vi "UDP广播.vi"(4 "接收间隔(5ms)":u32=5, 6 "发送间隔(25ms)":u32=25, 7 "文本控件":refnum<vi>, 8 "错误输入（无错误）":errorcluster, 10 "数据输入":string="www.usr.cn", 11 "端口或服务名称":u16=48899) -> (0 "error out":errorcluster caption="错误输出", 3 "接收":string[](array[string])=["192.168.1.221,D8B04CECA550,USR-C215,2.2.6", "192.168.1.220,ACCF2363AFF8,"])   [LabVIEW 2017]
uses:
  f306e6eb-da80-433f-8739-1ff3909e1865.vi
panel:
  out "发送次数":i32
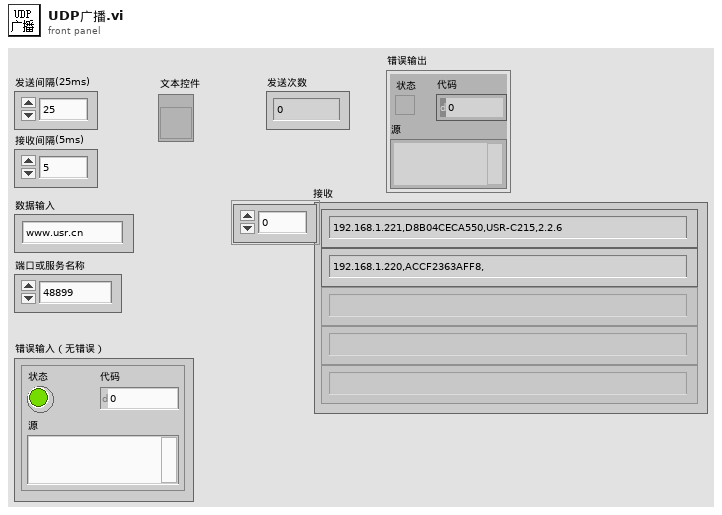
[diagram p1: front panel]
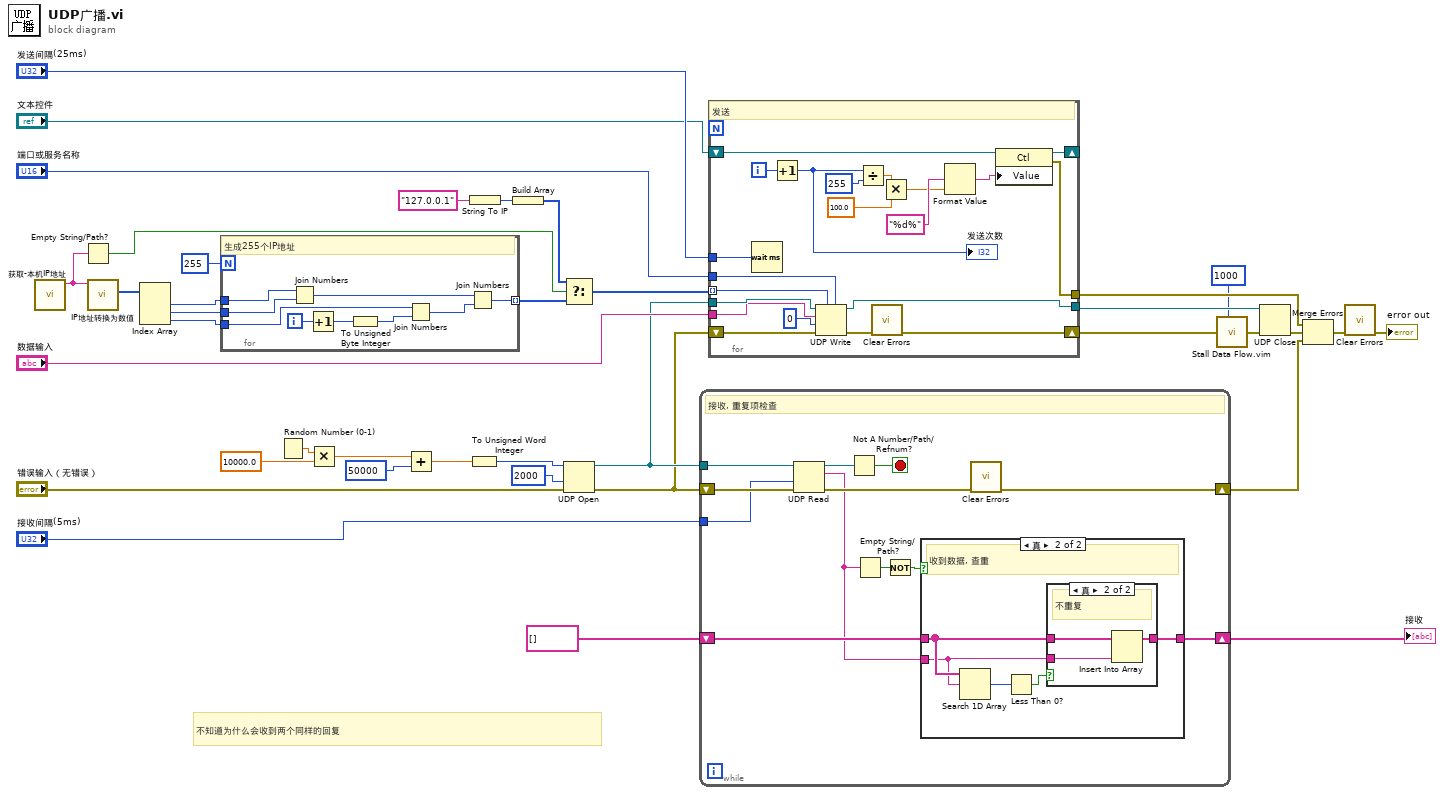
[diagram p0: block diagram]
diagram:
  # "不知道为什么会收到两个同样的回复"
  n1 = call "获取-本机IP地址.vi"() -> ("本机IP"=w27:string)  [unwired: 11 in]
  n2 = Empty String/Path?(string/path=w27) -> (empty?=w33:bool)
  n3 = call "IP地址转换为数值.vi"("IP地址"=w27) -> ("数组"=w38:u8[])  [unwired: 8 in, 2 out]
  n4 = Index Array(array=w38) -> (element #1=w36:u8, element #2=w35:u8, element #3=w34:u8)  [unwired: 3 in]
  n5 = for {
    N: 255 -> [_]
    tunnel: w36 -> [w44]
    tunnel: w35 -> [w43]
    tunnel: w34 -> [w42]
    tunnel: [w39] -> w29 mode=indexing
    i -> [w47]
    # "生成255个IP地址"
    n6 = Join Numbers(hi=w44, lo=w43) -> ((hi.lo)=w40:u16)
    n7 = Increment(x=w47) -> (x+1=w46:i32)
    n8 = To Unsigned Byte Integer(number=w46) -> (unsigned 8bit integer=w45:u8)
    n9 = Join Numbers(hi=w42, lo=w45) -> ((hi.lo)=w41:u16)
    n10 = Join Numbers(hi=w40, lo=w41) -> ((hi.lo)=w39:u32)
  }
  n11 = Random Number (0-1)() -> (number: 0 to 1=w20:dbl)
  n12 = Multiply(x=w20, y=10000.0) -> (x*y=w18:dbl)
  n13 = Add(x=w18, y=u16 50000 ("端口")) -> (x+y=w16:dbl)
  n14 = To Unsigned Word Integer(number=w16) -> (unsigned 16bit integer=w15:u16)
  n15 = String To IP(1:"127.0.0.1" ("名称")) -> (0:w31:u32)
  n16 = Build Array(w31) -> (w30:u32[])
  n17 = Select(t=w30, s=w33, f=w29) -> (s? t:f=w28:u32[])
  n18 = UDP Open(8:"错误输入（无错误）", 9:2000 ("超时毫秒(25000)"), 11:w15) -> (port=w22:refnum<k16>, 0:w21:errorcluster)  [unwired: 2 in, 1 out]
  n19 = while {
    tunnel: w22 -> [w59]
    shift-right: [w56] -> w11
    shift-left: w21 -> [w58]
    tunnel: "接收间隔(5ms)" -> [w52]
    shift-right: [w48] -> w1
    shift-left: string[] [] -> [w50]
    stop <- w53 stop-if-true
    # "接收, 重复项检查"
    n20 = UDP Read(connection ID=w59, timeout ms (25000)=w52, 8:w58) -> (data out=w49:string, error out=w55:errorcluster, 3:w54:refnum<k16>)  [unwired: 1 in, 2 out]
    n21 = Not A Number/Path/Refnum?(number/path/refnum=w54) -> (NaN/Path/Refnum?=w53:bool)
    n22 = Empty String/Path?(string/path=w49) -> (empty?=w57:bool)
    n23 = Not(x=w57) -> (.not. x?=w51:bool)
    n24 = case shown="真" w51 {
      tunnel: w50 -> [w60 w64]
      tunnel: w49 -> [_ w63]
      tunnel: [w60 w61] -> w48
      frame False {
        # "未收到数据"
      }
      frame True {
        # "收到数据, 查重"
        n25 = Search 1D Array(1D array=w64, element=w63) -> (index of element=w65:i32)  [unwired: 1 in]
        n26 = Less Than 0?(x=w65) -> (x < 0?=w62:bool)
        n27 = case shown="真" w62 {
          tunnel: w64 -> [w66 w69]
          tunnel: w63 -> [_ w68]
          tunnel: [w66 w67] -> w61
          frame False {
            # "重复, 不加"
          }
          frame True {
            # "不重复"
            n28 = Insert Into Array(array=w69, new element=w68) -> (w67:string[])  [unwired: 1 in]
          }
        }
      }
    }
    n29 = call <vilib>:"Clear Errors.vi"("error in (no error)"=w55) -> ("error out"=w56:errorcluster)  [unwired: 5 in, 1 out]
  }
  "接收" <- w1
  n30 = for {
    tunnel: w28 -> [w83] mode=indexing
    tunnel: "数据输入" -> [w89]
    tunnel: "端口或服务名称" -> [w87]
    shift-right: [w82] -> w9
    shift-left: w21 -> [w85]
    tunnel: w22 -> [w90]
    tunnel: [w88] -> w23
    tunnel: "发送间隔(25ms)" -> [w81]
    shift-right: [w78] -> _
    shift-left: "文本控件" -> [w79]
    tunnel: [w77] -> w7
    i -> [w80]
    # "发送"
    n31 = Wait (ms)(milliseconds to wait=w81) -> ()  [unwired: 1 out]
    n32 = Increment(x=w80) -> (x+1=w75:i32)
    "发送次数" <- w75
    n33 = UDP Write(address=w83, port or service name=w87, connection ID=w90, data in=w89, 8:w85, 9:0 ("超时毫秒(25000)")) -> (error out=w86:errorcluster, 3:w88:refnum<k16>)
    n34 = Divide(x=w75, y=255 ("x")) -> (x/y=w73:dbl)
    n35 = call <vilib>:"Clear Errors.vi"("error in (no error)"=w86) -> ("error out"=w82:errorcluster)  [unwired: 5 in, 1 out]
    n36 = Multiply(x=w73, y=100.0) -> (x*y=w71:dbl)
    n37 = Format Value(format string="%d%" ("格式字符串"), value (0)=w71) -> (output string=w72:string)  [unwired: 1 in]
    n38 = property class="Ctl"(reference=w79, "Value"=w72) -> (reference out=w78:refnum<vi>, error out=w77:errorcluster)  [unwired: 1 in]
  }
  n39 = call "Stall Data Flow.vim"("value in"=w9, "milliseconds to wait"=u32 1000) -> ("value out"=w13:errorcluster)  [unwired: 1 out]
  n40 = UDP Close(connection ID=w23, 8:w13) -> (error out=w10:errorcluster)  [unwired: 1 out]
  n41 = Merge Errors(w7, w10, w11) -> (w6:errorcluster)
  n42 = call <vilib>:"Clear Errors.vi"("error in (no error)"=w6) -> ("error out"=→"error out":errorcluster)  [unwired: 5 in, 1 out]
